vi "test Get VS Channel Handles and Messages.vi"(8 "error in (no error)":errorcluster) -> (0 "error out":errorcluster)   [LabVIEW 2020, in "Create Execution Unit.lvclass"]
uses:
  Create Execution Unit.lvclass
  <vilib>/addons/_JKI Toolkits/VI Tester/TestCase.llb/TestCase.lvclass
  Engine/Implementation/Execution Unit/Execution Unit.lvclass
  Scripting/AIM MIL-STD-1553 Scripting.lvlib
  Shared/Direction.ctl
  C:/Program Files (x86)/National Instruments/LabVIEW 2020/vi.lib/addons/_JKI Toolkits/VI Tester/TestCase.llb/TestCase.lvclass
panel:
  in  "TestCase in":refnum<class "Create Execution Unit.lvclass">
  out "TestCase out":refnum<class "Create Execution Unit.lvclass">
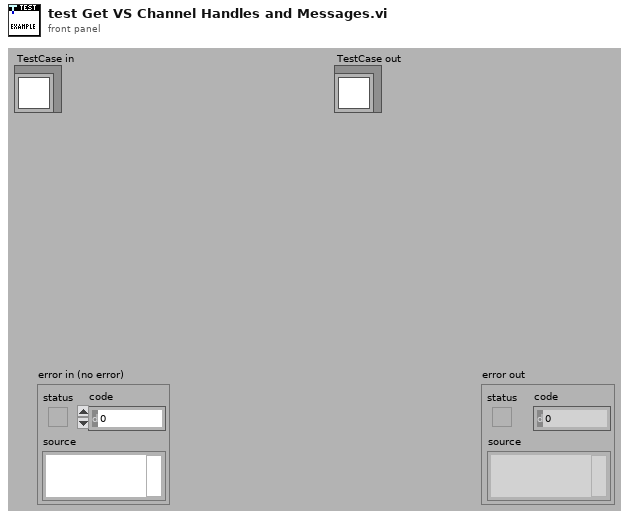
[diagram p1: front panel]
types:
  T1 = typedef "Direction.ctl" = enum16{"Rx", "Tx"}
  T2 = typedef "Custom Device API.lvlib/Custom Device Item Ref.ctl" = u64
  T3 = typedef "AIM MIL-STD-1553 Engine.lvlib/Custom Device.lvlib/Compiled Message.ctl" = cluster{"Message Section Handle":T2, "First Parameter Index":i32, "Parameter Channel Handles":T2[], "Direction":T1, "Parameters":T4[], "Receiving RT Address":u8, "Receiving RT Sub-address":u8, "Transmitting RT Address":u8, "Transmitting RT Sub-address":u8, "Word Count":u8, "Buffer Type":enum16{"unknown", "BC Message Buffer", "RT Message Buffer"}, "Buffer ID":u16, "Terminal Type":enum16{"Bus Controller", "Remote Terminal"}, "Timestamp Enabled":bool, "Timestamp Channel Handle":T2}
  T4 = typedef "Parameter Definition.ctl" = cluster{"start index":i32, "size (bits)":i32, "encoding":enum16{"BNR", "BCD", "Discrete"}, "signed":bool, "multiplier":dbl, "offset":dbl}
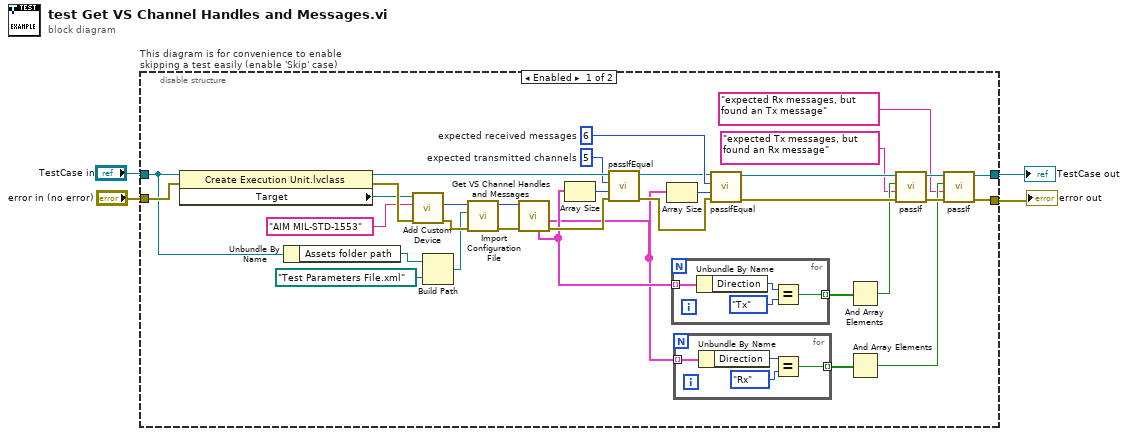
[diagram p0: block diagram]
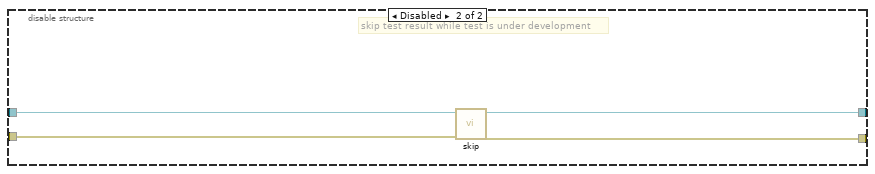
[diagram p2: hidden frame]
diagram:
  n1 = disable-structure "This diagram is for convenience to enable skipping a test easily (enable 'Skip' case)" shown="Enabled" {
    disable-tunnel: "TestCase in" -> [w29 w50]
    disable-tunnel: [w13 w48] -> w1
    disable-tunnel: [w12 w49] -> w3
    disable-tunnel: "error in (no error)" -> [w30 w47]
    frame Enabled {
      w22 = 6  # expected received messages
      w24 = 5  # expected transmitted channels
      n2 = property class="Create Execution Unit.lvclass"(reference=w29, error in=w30) -> (reference out=w26:refnum<class "Create Execution Unit.lvclass">, error out=w33:errorcluster, "Target"=w32:refnum<k24>)
      n3 = Unbundle By Name(w29) -> ("Assets folder path"=w34:path)
      n4 = call "Add Custom Device.vi"("error in"=w33, "custom device name"="AIM MIL-STD-1553" ("name"), "target"=w32) -> ("error out"=w38:errorcluster, "custom device"=w37:T2)  [unwired: 6 in, 1 out]
      n5 = Build Path(base path=w34, name or relative path=path "Test Parameters File.xml") -> (appended path=w36:path)
      n6 = call "Import Configuration File.vi"("error in"=w38, "parameters configuration file path"=w36, "custom device"=w37) -> ("error out"=w27:errorcluster, "custom device out"=w28:T2)  [unwired: 7 in]
      n7 = call "Get VS Channel Handles and Messages.vi"("error in"=w27, "custom device ref"=w28) -> ("error out"=w20:errorcluster, "received messages and subaddresses"=w5:T3[], "transmitted messages and subaddresses"=w18:T3[])  [unwired: 2 in, 5 out]
      n8 = Array Size(array=w18) -> (size(s)=w25:i32)
      n9 = call-dynamic "passIfEqual.vi"("error in (no error)"=w20, "y"=w25, "x"=w24, "TestCase in"=w26) -> ("error out"=w19:errorcluster, "TestCase out"=w21:refnum<class "Create Execution Unit.lvclass">)  [unwired: 6 in]
      n10 = Array Size(array=w5) -> (size(s)=w23:i32)
      n11 = for {
        tunnel: w18 -> [w46] mode=indexing
        tunnel: [w43] -> w11 mode=indexing
        n12 = Unbundle By Name(w46) -> ("Direction"=w44:T1)
        n13 = Equal?(x=w44, y=Direction."Tx" ("Direction")) -> (x = y?=w43:bool)
      }
      n14 = for {
        tunnel: w5 -> [w42] mode=indexing
        tunnel: [w39] -> w9 mode=indexing
        n15 = Unbundle By Name(w42) -> ("Direction"=w40:T1)
        n16 = Equal?(x=w40, y=Direction."Rx" ("Direction")) -> (x = y?=w39:bool)
      }
      n17 = call-dynamic "passIfEqual.vi"("error in (no error)"=w19, "y"=w23, "x"=w22, "TestCase in"=w21) -> ("error out"=w17:errorcluster, "TestCase out"=w16:refnum<class "Create Execution Unit.lvclass">)  [unwired: 6 in]
      n18 = And Array Elements(Boolean array=w11) -> (logical AND=w10:bool)
      n19 = And Array Elements(Boolean array=w9) -> (logical AND=w8:bool)
      n20 = call-dynamic "passIf.vi"("error in (no error)"=w17, "message (\"\")"="expected Tx messages, but found an Rx message" ("message (\"\")"), "pass"=w10, "TestCase in"=w16) -> ("error out"=w14:errorcluster, "TestCase out"=w15:refnum<class "Create Execution Unit.lvclass">)  [unwired: 6 in]
      n21 = call-dynamic "passIf.vi"("error in (no error)"=w14, "message (\"\")"="expected Rx messages, but found an Tx message" ("message (\"\")"), "pass"=w8, "TestCase in"=w15) -> ("error out"=w12:errorcluster, "TestCase out"=w13:refnum<class "Create Execution Unit.lvclass">)  [unwired: 6 in]
    }
    frame Disabled {
      # "skip test result while test is under development"
      n22 = call <vilib>:"skip.vi"("error in (no error)"=w47, "TestCase in"=w50) -> ("error out"=w49:errorcluster, "TestCase out"=w48:refnum<class "Create Execution Unit.lvclass">)  [unwired: 8 in]
    }
  }
  "error out" <- w3
  "TestCase out" <- w1
